vi "Read Raw.vi"(8 "error in (no error)":errorcluster, 11 "AODAcq in":refnum<class "AODAcq.lvclass">) -> (0 "error out":errorcluster, 3 "AODAcq out":refnum<class "AODAcq.lvclass">)   [LabVIEW 2014, in "AODAcq.lvclass"]
uses:
  AODAcq.lvclass
  AODAcq.lvclass/AODAcq.ctl
  <vilib>/Utility/error.llb/Error Cluster From Error Code.vi
  <vilib>/rvi/errors/niLvFpgaAdjustHostInterfaceError.vi
  HDF5Tools/LabView/Append To Dataset 1D Integer.vi
  <vilib>/rvi/interface/nirviMethod/nirviMethod.xnode
  FPGA_Control/AODRef.ctl
  FPGA Bitfiles/AodScanner_FPGATarget_AODControl(FPGA)_TyJc9yYmyGA.lvbitx
  <vilib>/rvi/errors/niLvFpgaMergeErrorWithErrorCode.vi
  HDF5Tools/LabView/HDF5Tools.lvlib
  <vilib>/FPGAPlugInAG/PXIe-7965R/niLvFpga_ReadFifo_PXIe-7965R.vi
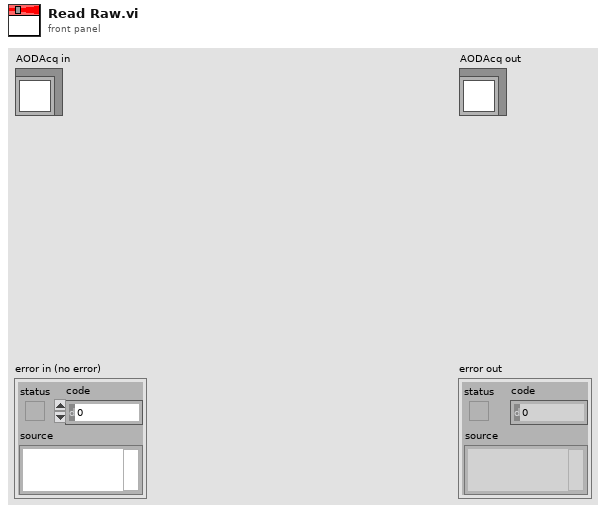
[diagram p1: front panel]
types:
  T1 = typedef "AODRef.ctl" = refnum<k20>
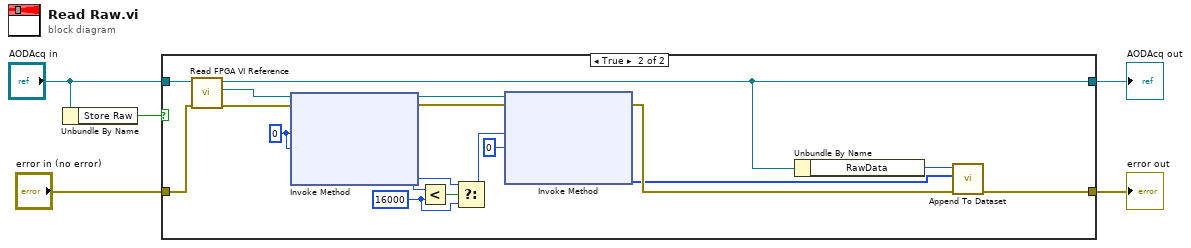
[diagram p0: block diagram]
diagram:
  n1 = Unbundle By Name("AODAcq in") -> ("Store Raw"=w5:bool)
  n2 = case shown="True" w5 {
    tunnel: [w7 w15] -> w2
    tunnel: "AODAcq in" -> [w7 w24]
    tunnel: "error in (no error)" -> [w6 w18]
    tunnel: [w6 w14] -> w1
    frame False {
    }
    frame True {
      w12 = u32 16000 ("y")
      w23 = u32 0 ("Number of Elements")
      n3 = call-dynamic "Read FPGA VI Reference.vi"("error in (no error)"=w18, "AODAcq in"=w24) -> ("error out"=w19:errorcluster, "FPGA VI Reference"=w17:T1, "AODAcq out"=w15:refnum<class "AODAcq.lvclass">)  [unwired: 7 in]
      n4 = xnode "Invoke Method"("FPGA VI Reference In"=w17, "error in"=w19, "Number of Elements"=w23, "Timeout (ms)"=w23) -> ("FPGA VI Reference Out"=w22:T1, "error out"=w21:errorcluster, "Elements Remaining"=w11:u32)  [unwired: 1 out]
      n5 = Less?(x=w11, y=w12) -> (x < y?=w13:bool)
      n6 = Select(t=w11, s=w13, f=w12) -> (s? t:f=w10:u32)
      n7 = xnode "Invoke Method"("FPGA VI Reference In"=w22, "error in"=w21, "Number of Elements"=w10, "Timeout (ms)"=0) -> ("error out"=w16:errorcluster, "Data"=w9:i16[])  [unwired: 2 out]
      n8 = Unbundle By Name(w15) -> ("RawData"=w8:i32)
      n9 = call-poly "Append To Dataset.vi"("error in (no error)"=w16, "data"=w9, "Dataset id in"=w8) -> ("Error out"=w14:errorcluster)  [unwired: 7 in, 1 out]
    }
  }
  "error out" <- w1
  "AODAcq out" <- w2
